vi "Init Power Supply.vi"(0 "Power Supply Address":refnum<visa-resource-name>, 1 "PS Control References Cluster":T1, 2 "Power Supply Config on Startup":enum16{"PC->Power Supply", "Power Supply->PC"}(ring), 3 "ResetPS Settings":bool, 4 "Power Supply Model":T2(ring)=enum."Keithley 24XX", 5 "error in":errorcluster) -> (6 "VISA resource name out":refnum<visa-resource-name>, 7 "Instrument Name":string, 8 "error out":errorcluster)   [LabVIEW 2020]
uses:
  <instrlib>/Keithley 24XX/Keithley 24XX.lvlib
panel:
  in  "Timeout (ms)":i32=2000
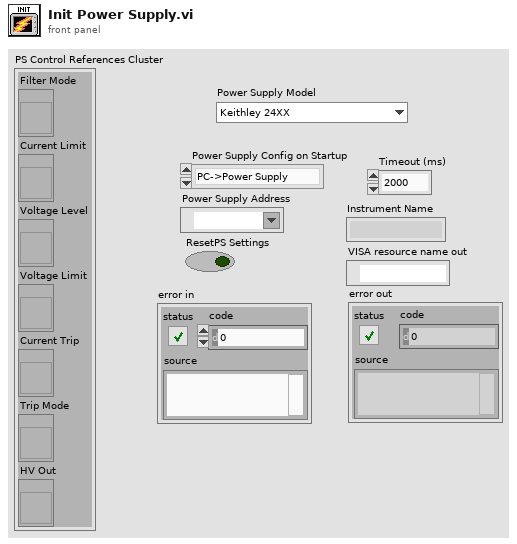
[diagram p1: front panel]
types:
  T1 = cluster{"Filter Mode":refnum<vi>, "Current Limit":refnum<vi>, "Voltage Level":refnum<vi>, "Voltage Limit":refnum<vi>, "Current Trip":refnum<vi>, "Trip Mode":refnum<vi>, "HV Out":refnum<vi>}
  T2 = enum16{"Keithley 248", "Keithley 237", "Keithley 24XX"}
  T3 = cluster{"Min V":dbl, "Max V":dbl, "Min I":dbl, "Max I":dbl}
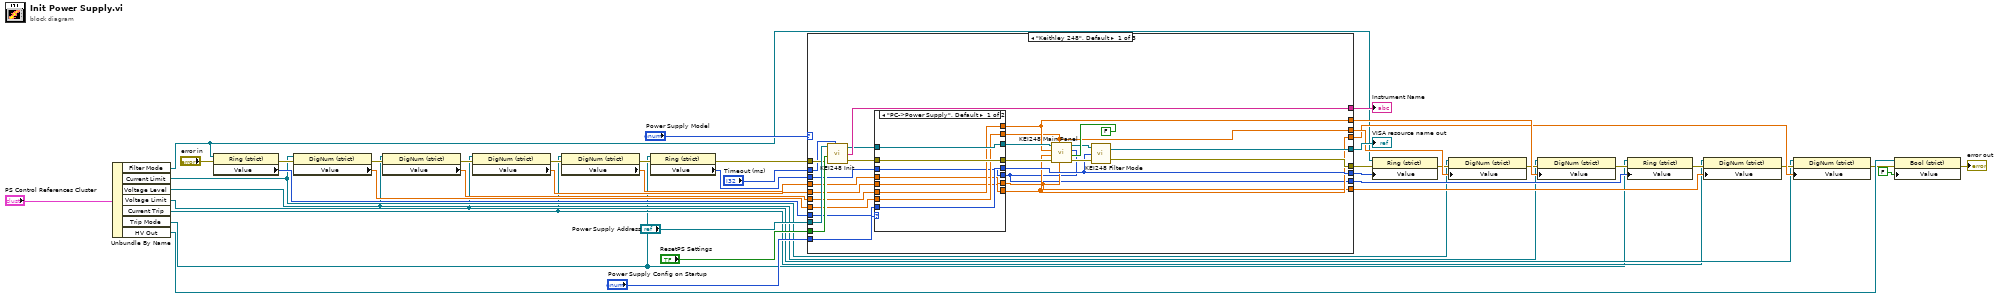
[diagram p0: block diagram]
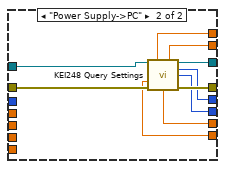
[diagram p2: hidden frame]
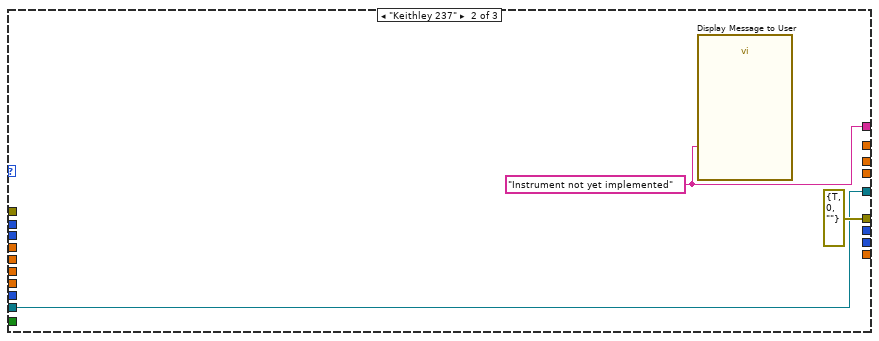
[diagram p3: hidden frame]
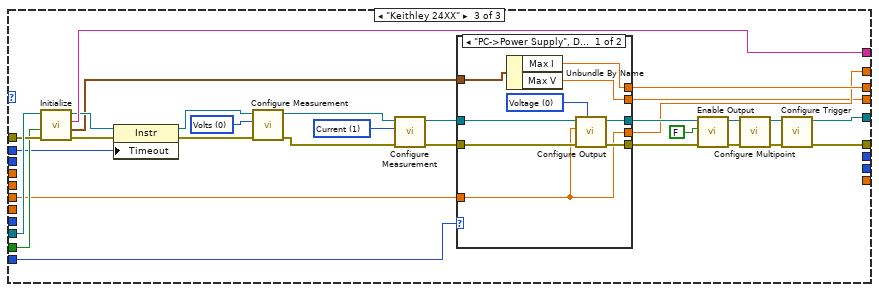
[diagram p4: hidden frame]
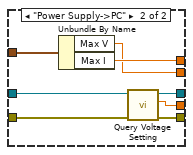
[diagram p5: hidden frame]
diagram:
  n1 = Unbundle By Name("PS Control References Cluster") -> ("Filter Mode"=w11:refnum<vi>, "Current Limit"=w10:refnum<vi>, "Voltage Level"=w9:refnum<vi>, "Voltage Limit"=w8:refnum<vi>, "Current Trip"=w7:refnum<vi>, "Trip Mode"=w6:refnum<vi>, "HV Out"=w4:refnum<vi>)
  n2 = property class="Ring (strict)"(reference=w11, error in="error in") -> (error out=w25:errorcluster, "Value"=w20:u16)  [unwired: 1 out]
  n3 = property class="DigNum (strict)"(reference=w10, error in=w25) -> (error out=w24:errorcluster, "Value"=w19:dbl)  [unwired: 1 out]
  n4 = property class="DigNum (strict)"(reference=w9, error in=w24) -> (error out=w23:errorcluster, "Value"=w18:sgl)  [unwired: 1 out]
  n5 = property class="DigNum (strict)"(reference=w8, error in=w23) -> (error out=w22:errorcluster, "Value"=w17:dbl)  [unwired: 1 out]
  n6 = property class="DigNum (strict)"(reference=w7, error in=w22) -> (error out=w21:errorcluster, "Value"=w16:dbl)  [unwired: 1 out]
  n7 = property class="Ring (strict)"(reference=w6, error in=w21) -> (error out=w13:errorcluster, "Value"=w15:u16)  [unwired: 1 out]
  n8 = case shown="\"Keithley 248\", Default" "Power Supply Model" {
    tunnel: "Power Supply Address" -> [w70 w89 w121]
    tunnel: [w69 w90 w118] -> w40
    tunnel: [w58 w89 w104] -> w39
    tunnel: [w57 errorcluster {"status"=TRUE, "code"=0, "source"=""} ("error constant") w103] -> w31
    tunnel: "ResetPS Settings" -> [w68 _ w119]
    tunnel: w13 -> [w67 _ w120]
    tunnel: "Power Supply Config on Startup" -> [w61 _ w102]
    tunnel: "Timeout (ms)" -> [w56 _ w92]
    tunnel: [w55 _ _] -> w38
    tunnel: [w54 _ w94] -> w37
    tunnel: [w53 _ w96] -> w36
    tunnel: [w52 _ w93] -> w35
    tunnel: [w51 _ _] -> w34
    tunnel: [w50 _ _] -> w33
    tunnel: w20 -> [w49 _ _]
    tunnel: w19 -> [w48 _ _]
    tunnel: w18 -> [w47 _ w95]
    tunnel: w17 -> [w46 _ _]
    tunnel: w16 -> [w45 _ _]
    tunnel: w15 -> [w44 _ _]
    frame "Keithley 248", Default {
      n9 = call <instrlib>:"KEI248 Init.vi"("VISA resource name"=w70, "Reset (False)"=w68, "error in"=w67, "VISA Timeout (10s)"=w56) -> ("VISA resource name out"=w63:refnum<visa-resource-name>, "Instrument Name"=w69:string, "error out"=w62:errorcluster)  [unwired: 1 in]
      n10 = case shown="\"PC->Power Supply\", Default" w61 {
        tunnel: [w78 w88] -> w66
        tunnel: [w77 w87] -> w65
        tunnel: [w71 w80] -> w50
        tunnel: [w75 w82] -> w53
        tunnel: [w72 w81] -> w51
        tunnel: [w73 w83] -> w52
        tunnel: [w74 w84] -> w54
        tunnel: w63 -> [w78 w86]
        tunnel: w62 -> [w77 w85]
        tunnel: [w76 w79] -> w55
        tunnel: w49 -> [w76 _]
        tunnel: w48 -> [w75 _]
        tunnel: w47 -> [w74 _]
        tunnel: w46 -> [w73 _]
        tunnel: w45 -> [w72 _]
        tunnel: w44 -> [w71 _]
        frame "PC->Power Supply", Default {
        }
        frame "Power Supply->PC" {
          n11 = call "KEI248 Query Settings"("VISA resource name"=w86, "error in (no error)"=w85) -> ("Voltage Setting"=w84:dbl, "Current Limit"=w82:dbl, "VISA resource name out"=w88:refnum<visa-resource-name>, "Filter Mode"=w79:i8, "Trip Reset Mode"=w80:i8, "Voltage Limit"=w83:dbl, "Current Trip"=w81:dbl, "error out"=w87:errorcluster)  [unwired: 3 in, 3 out]
        }
      }
      n12 = call "KEI248 Main Panel"("Output Switch"=FALSE, "Trip Mode"=w50, "Current Trip"=w51, "Current Limit"=w53, "error in"=w65, "Voltage Limit"=w52, "Voltage Setting"=w54, "VISA resource name"=w66) -> ("error out"=w59:errorcluster, "VISA resource name out"=w60:refnum<visa-resource-name>)
      n13 = call "KEI248 Filter Mode"("error in"=w59, "Filter Mode"=w55, "VISA resource name"=w60) -> ("error out"=w57:errorcluster, "VISA resource name out"=w58:refnum<visa-resource-name>)
    }
    frame "Keithley 237" {
      w90 = "Instrument not yet implemented" ("Message")
      n14 = call "Display Message to User"("Message"=w90) -> ()  [unwired: 9 in, 2 out]
    }
    frame "Keithley 24XX" {
      w109 = u16 0 items=["Volts", "Current", "Resistance"] ("Function (0: Volts)")
      w108 = u16 1 items=["Volts", "Current", "Resistance"] ("Function (0: Volts)")
      n15 = call <instrlib>:"Initialize.vi"("error in (no error)"=w120, "Reset (True)"=w119, "VISA resource name"=w121) -> ("error out"=w116:errorcluster, "Source Range"=w101:T3, "Instrument Name"=w118:string, "VISA resource name out"=w117:refnum<visa-resource-name>)  [unwired: 5 in]
      n16 = property class="Instr"(reference=w117, error in=w116, "Timeout"=w92) -> (reference out=w106:refnum<visa-resource-name>, error out=w105:errorcluster)
      n17 = call <instrlib>:"Configure Measurement.vi"("error in (no error)"=w105, "Function (0: Volts)"=w109, "VISA resource name"=w106) -> ("error out"=w111:errorcluster, "VISA resource name out"=w110:refnum<visa-resource-name>)  [unwired: 7 in]
      n18 = call <instrlib>:"Configure Measurement.vi"("error in (no error)"=w111, "Function (0: Volts)"=w108, "VISA resource name"=w110) -> ("error out"=w100:errorcluster, "VISA resource name out"=w99:refnum<visa-resource-name>)  [unwired: 7 in]
      n19 = case shown="\"PC->Power Supply\", Default" w102 {
        tunnel: w101 -> [w125 w138]
        tunnel: w100 -> [w130 w136]
        tunnel: w99 -> [w129 w137]
        tunnel: [w128 w135] -> w98
        tunnel: [w127 w134] -> w97
        tunnel: [w124 w133] -> w96
        tunnel: w95 -> [w123 _]
        tunnel: [w123 w132] -> w94
        tunnel: [w122 w131] -> w93
        frame "PC->Power Supply", Default {
          w126 = u16 0 items=["Voltage", "Current"] ("Source Mode  (0: Voltage)")
          n20 = Unbundle By Name(w125) -> ("Max I"=w124:dbl, "Max V"=w122:dbl)
          n21 = call <instrlib>:"Configure Output.vi"("Source Mode  (0: Voltage)"=w126, "error in (no error)"=w130, "Output Level (0)"=w123, "VISA resource name"=w129) -> ("error out"=w128:errorcluster, "VISA resource name out"=w127:refnum<visa-resource-name>)  [unwired: 6 in]
        }
        frame "Power Supply->PC" {
          n22 = Unbundle By Name(w138) -> ("Max V"=w131:dbl, "Max I"=w133:dbl)
          n23 = call <instrlib>:"Query Voltage Setting.vi"("error in (no error)"=w136, "VISA resource name"=w137) -> ("error out"=w135:errorcluster, "Voltage"=w132:dbl, "VISA resource name out"=w134:refnum<visa-resource-name>)  [unwired: 7 in]
        }
      }
      n24 = call <instrlib>:"Enable Output.vi"("error in (no error)"=w98, "Enable Output (T: Enable)"=FALSE, "VISA resource name"=w97) -> ("error out"=w113:errorcluster, "VISA resource name out"=w115:refnum<visa-resource-name>)  [unwired: 7 in]
      n25 = call <instrlib>:"Configure Multipoint.vi"("error in (no error)"=w113, "VISA resource name"=w115) -> ("error out"=w114:errorcluster, "VISA resource name out"=w112:refnum<visa-resource-name>)  [unwired: 8 in]
      n26 = call <instrlib>:"Configure Trigger.vi"("error in (no error)"=w114, "VISA resource name"=w112) -> ("error out"=w103:errorcluster, "VISA resource name out"=w104:refnum<visa-resource-name>)  [unwired: 8 in]
    }
  }
  "Instrument Name" <- w40
  "VISA resource name out" <- w39
  n27 = property class="Ring (strict)"(reference=w11, error in=w31, "Value"=w38) -> (error out=w30:errorcluster)  [unwired: 1 out]
  n28 = property class="DigNum (strict)"(reference=w10, error in=w30, "Value"=w36) -> (error out=w29:errorcluster)  [unwired: 1 out]
  n29 = property class="DigNum (strict)"(reference=w9, error in=w29, "Value"=w37) -> (error out=w28:errorcluster)  [unwired: 1 out]
  n30 = property class="Ring (strict)"(reference=w6, error in=w28, "Value"=w33) -> (error out=w27:errorcluster)  [unwired: 1 out]
  n31 = property class="DigNum (strict)"(reference=w7, error in=w27, "Value"=w34) -> (error out=w26:errorcluster)  [unwired: 1 out]
  n32 = property class="DigNum (strict)"(reference=w8, error in=w26, "Value"=w35) -> (error out=w2:errorcluster)  [unwired: 1 out]
  n33 = property class="Bool (strict)"(reference=w4, error in=w2, "Value"=FALSE) -> (error out=→"error out":errorcluster)  [unwired: 1 out]
